vi "Initialize From File.vi"(0 "Component in":refnum<class "Component.lvclass">) -> (4 "Component out":refnum<class "Component.lvclass">)   [LabVIEW 2017, in "CL_G3_VIComponentBuilder.lvlib" / "Component.lvclass"]
doc: "Initializes the class from the configuration file."
uses:
  Component.lvclass
  Component.lvclass/Component.ctl
  Exports/Exports/Export.lvclass/Export.ctl
  Accessors/Read Component Config File.vi
  Exports/Exports/Accessors/Read Export Operation Errors.vi
  Exports/Exports/Accessors/Read unique Name.vi
  Exports/Exports/Accessors/Write Owning Component's Product Name.vi
  Exports/Exports/Accessors/Write Owning Component's Unique Name.vi
  Accessors/Read Component Path.vi
  Accessors/Read Product Name.vi
  Accessors/Read Unique Name.vi
  Accessors/Write Component Operations Errors.vi
  Accessors/Read Component Operations Errors.vi
  Accessors/Write Unique Name.vi
  Accessors/Write Product Name.vi
  <vilib>/ErrorRing/Error Ring.xnode
  <vilib>/Utility/config.llb/NI_LVConfig.lvlib
  Exports/Exports/Export.lvclass
  CL_G3_VIComponentBuilder.lvlib
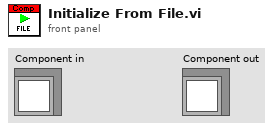
[diagram p1: front panel]
types:
  T1 = cluster{"Product Name":string, "Unique Name":string, "Exports":cluster{"Export Definition File":path}[]}
  T2 = typedef "NI_LVConfig.lvlib/Config Data RefNum.ctl" = refnum<k1>
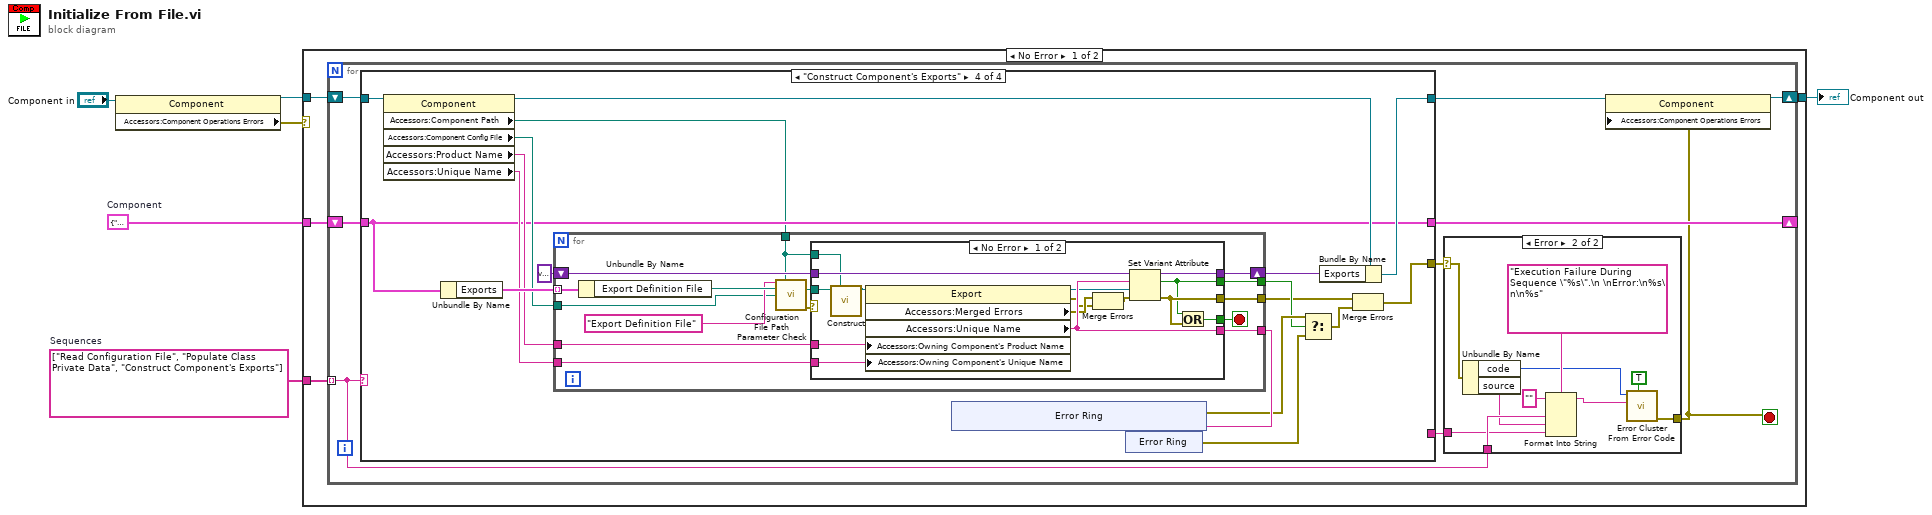
[diagram p0: block diagram]
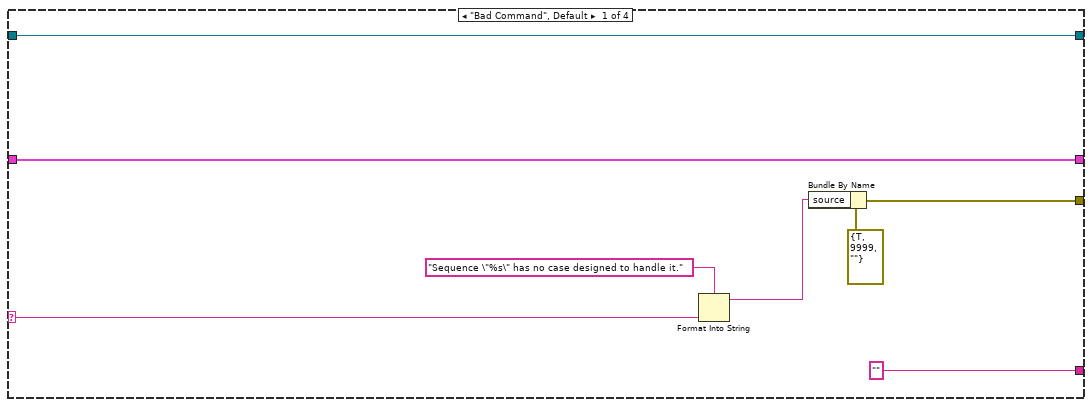
[diagram p3: hidden frame]
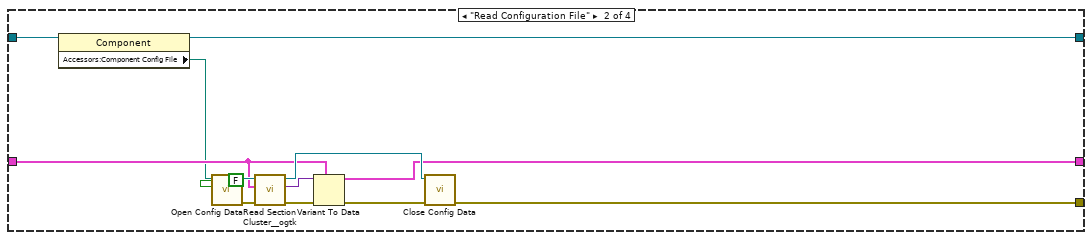
[diagram p4: hidden frame]
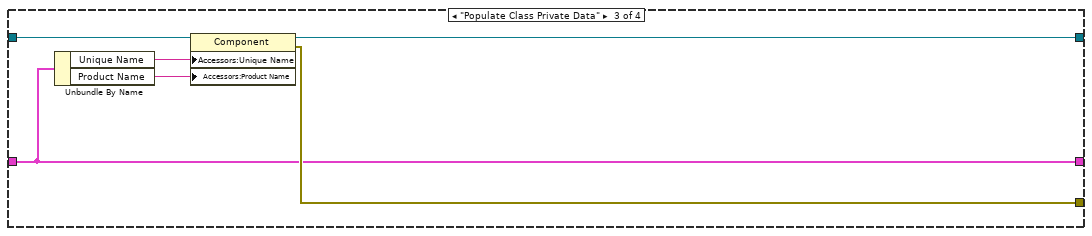
[diagram p5: hidden frame]
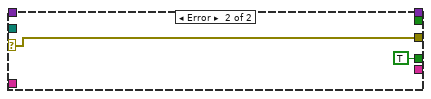
[diagram p6: hidden frame]
diagram:
  w4 = T1 {"Product Name"="", "Unique Name"="", "Exports"=[]}  # Component
  w6 = string[] ["Read Configuration File", "Populate Class Private Data", "Construct Component's Exports"]  # Sequences
  n1 = property class="Component"(reference="Component in") -> (reference out=w1:refnum<class "Component.lvclass">, "Accessors:Component Operations Errors"=w2:errorcluster)  [unwired: 1 in, 1 out]
  n2 = case shown="No Error" w2 {
    tunnel: w6 -> [w10 _]
    tunnel: w1 -> [w9 w116]
    tunnel: w4 -> [w8 _]
    tunnel: [w7 w116] -> w3
    frame No Error {
      n3 = for {
        tunnel: w10 -> [w18] mode=indexing
        shift-right: [w14] -> w7
        shift-left: w9 -> [w19]
        shift-right: [w15] -> _
        shift-left: w8 -> [w16]
        stop <- w11 stop-if-true
        n4 = case shown="\"Construct Component's Exports\"" w18 {
          selector: w18 -> [w33 _ _ _]
          tunnel: w19 -> [w38 w51 w57 w75]
          tunnel: [w38 w43 w56 w62] -> w13
          tunnel: [w35 w39 w53 w60] -> w12
          tunnel: ["" ("Accessors:Name") _ _ _] -> w17
          tunnel: w16 -> [w31 w41 w52 w61]
          tunnel: [w31 w42 w52 w61] -> w15
          frame "Bad Command", Default {
            n5 = Format Into String(format string="Sequence \"%s\" has no case designed to handle it.", w33) -> (resulting string=w32:string)  [unwired: 2 in, 1 out]
            n6 = Bundle By Name(cluster=errorcluster {"status"=TRUE, "code"=9999, "source"=""} ("error out"), "source"=w32) -> (w35:errorcluster)
          }
          frame "Read Configuration File" {
            n7 = property class="Component"(reference=w51) -> (reference out=w43:refnum<class "Component.lvclass">, "Accessors:Component Config File"=w40:path)  [unwired: 1 in, 1 out]
            n8 = call <vilib>:"Open Config Data.vi"("create file if necessary (T)"=FALSE, "configuration file path"=w40) -> ("error out"=w44:errorcluster, "refnum"=w48:T2)  [unwired: 7 in, 1 out]
            n9 = call <userlib>:"Read Section Cluster__ogtk.vi"("error in (no error)"=w44, "Section Formatted Cluster Type"=w41, "refnum"=w48) -> ("error out"=w46:errorcluster, "Section Formatted Cluster"=w49:variant, "dup refnum"=w47:T2)  [unwired: 4 in, 2 out]
            n10 = Variant To Data(error in=w46, type=w41, Variant=w49) -> (data=w42:T1, error out=w45:errorcluster)
            n11 = call <vilib>:"Close Config Data.vi"("error in (no error)"=w45, "refnum"=w47) -> ("error out"=w39:errorcluster)  [unwired: 8 in, 1 out]
          }
          frame "Populate Class Private Data" {
            n12 = Unbundle By Name(w52) -> ("Unique Name"=w55:string, "Product Name"=w54:string)
            n13 = property class="Component"(reference=w57, "Accessors:Unique Name"=w55, "Accessors:Product Name"=w54) -> (reference out=w56:refnum<class "Component.lvclass">, error out=w53:errorcluster)  [unwired: 1 in]
          }
          frame "Construct Component's Exports" {
            n14 = property class="Component"(reference=w75) -> (reference out=w63:refnum<class "Component.lvclass">, "Accessors:Component Path"=w58:path, "Accessors:Component Config File"=w64:path, "Accessors:Product Name"=w66:string, "Accessors:Unique Name"=w65:string)  [unwired: 1 in, 1 out]
            n15 = Unbundle By Name(w61) -> ("Exports"=w67:cluster{"Export Definition File":path}[])
            n16 = for {
              shift-right: [w98] -> w68
              shift-left: variant -> [w97]
              tunnel: w67 -> [w96] mode=indexing
              tunnel: [w95] -> w73
              tunnel: [w91] -> w71
              tunnel: w65 -> [w94]
              tunnel: w66 -> [w93]
              tunnel: [w92] -> w69
              tunnel: w64 -> [w85]
              tunnel: w58 -> [w84]
              stop <- w90 stop-if-true
              n17 = Unbundle By Name(w96) -> ("Export Definition File"=w89:path)
              n18 = call "Configuration File Path Parameter Check.vi"("Parameter Name"="Export Definition File", "Component Root Path"=w84, "Specified Path in Configuration File"=w89, "Configuration File Path"=w85) -> ("dup Specified Path in Configuration File"=w88:path, "error out"=w86:errorcluster)  [unwired: 9 in, 1 out]
              n19 = case shown="No Error" w86 {
                selector: w86 -> [_ w114]
                tunnel: [w112 _] -> w98
                tunnel: w97 -> [w111 _]
                tunnel: [w110 _] -> w95
                tunnel: w94 -> [w109 _]
                tunnel: w93 -> [w108 _]
                tunnel: [w107 w114] -> w92
                tunnel: [w106 _] -> w91
                tunnel: [w105 TRUE] -> w90
                tunnel: w88 -> [w104 _]
                tunnel: w84 -> [w99 _]
                frame No Error {
                  n20 = call "Construct.vi"("Export Config File"=w104, "Component Root Path"=w99) -> ("Export Out"=w113:refnum<class "Export.lvclass">)  [unwired: 13 in]
                  n21 = property class="Export"(reference=w113, "Accessors:Owning Component's Product Name"=w108, "Accessors:Owning Component's Unique Name"=w109) -> (reference out=w103:refnum<class "Export.lvclass">, error out=w100:errorcluster, "Accessors:Merged Errors"=w101:errorcluster, "Accessors:Unique Name"=w110:string)  [unwired: 1 in]
                  n22 = Merge Errors(w101, w100) -> (w102:errorcluster)
                  n23 = Set Variant Attribute(Variant=w111, name=w110, value=w103, error in=w102) -> (Variant out=w112:variant, replaced=w106:bool, error out=w107:errorcluster)
                  n24 = Or(x=w106, y=w107) -> (x .or. y?=w105:bool)
                }
                frame Error {
                }
              }
            }
            n25 = xnode "Error Ring"("parameter 0"=w73) -> ("error out"=w72:errorcluster)
            n26 = xnode "Error Ring"() -> ("error out"=w59:errorcluster)
            n27 = Select(t=w72, s=w71, f=w59) -> (s? t:f=w70:errorcluster)
            n28 = Bundle By Name(cluster=w63, "Exports"=w68) -> (w62:refnum<class "Component.lvclass">)
            n29 = Merge Errors(w69, w70) -> (w60:errorcluster)
          }
        }
        n30 = case shown="Error" w12 {
          selector: w12 -> [w20 w24]
          tunnel: [w20 w29] -> w11
          tunnel: w18 -> [_ w27]
          tunnel: w17 -> [_ w22]
          frame No Error {
          }
          frame Error {
            n31 = Unbundle By Name(w24) -> ("code"=w21:i32, "source"=w23:string)
            n32 = Format Into String(format string="Execution Failure During Sequence \"%s\".\n \nError:\n%s\n\n%s" ("error message (\"\")"), initial string="", w27, w23, w22) -> (resulting string=w28:string)  [unwired: 1 in, 1 out]
            n33 = call <vilib>:"Error Cluster From Error Code.vi"("show call chain? (False)"=TRUE, "error message (\"\")"=w28, "error code (0)"=w21) -> ("error out"=w29:errorcluster)  [unwired: 6 in]
          }
        }
        n34 = property class="Component"(reference=w13, "Accessors:Component Operations Errors"=w11) -> (reference out=w14:refnum<class "Component.lvclass">)  [unwired: 1 in, 1 out]
      }
    }
    frame Error {
    }
  }
  "Component out" <- w3
